vi "_ParseVIFunc.vi"(11 "string":string="VIB(sin(x)+2,VIA(x,y), VIB(z))") -> (0 "valid":bool=TRUE, 2 "Array of Strings":string[](array[string])=["sin(x)+2", "VIA(x", "y)", " VIB(z)"], 3 "before substring":string="VIB")   [LabVIEW 2017]
uses:
  <userlib>/_NEVSTOP/Communicable State Machine(CSM)/Communicable State Machine.lvlib
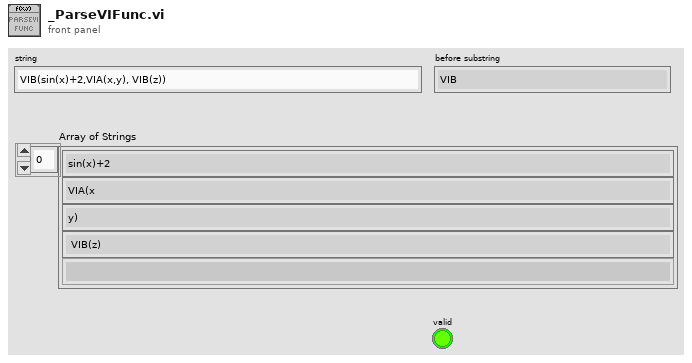
[diagram p1: front panel]
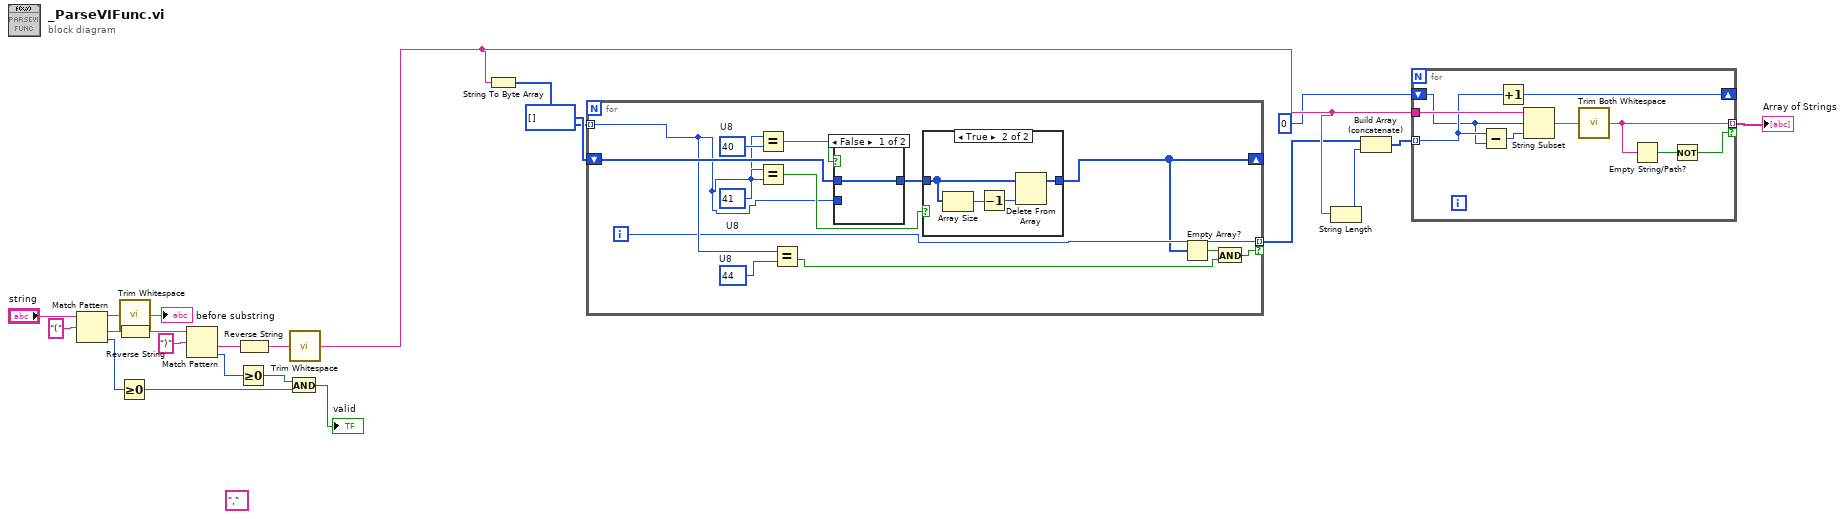
[diagram p0: block diagram]
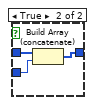
[diagram p3: hidden frame]
diagram:
  (unwired) "," ("regular expression")
  n1 = Match Pattern(string="string", regular expression="(") -> (before substring=w21:string, after substring=w19:string, offset past match=w17:i32)  [unwired: 1 in, 1 out]
  n2 = Greater Or Equal To 0?(x=w17) -> (x >= 0?=w14:bool)
  n3 = call <vilib>:"Trim Whitespace.vi"("string"=w21) -> ("trimmed string"=→"before substring":string)  [unwired: 1 in]
  n4 = Reverse String(1:w19) -> (0:w12:string)
  n5 = Match Pattern(string=w12, regular expression=")") -> (after substring=w11:string, offset past match=w16:i32)  [unwired: 1 in, 2 out]
  n6 = Greater Or Equal To 0?(x=w16) -> (x >= 0?=w15:bool)
  n7 = Reverse String(1:w11) -> (0:w10:string)
  n8 = And(x=w15, y=w14) -> (x .and. y?=→"valid":bool)
  n9 = call <vilib>:"Trim Whitespace.vi"("string"=w10) -> ("trimmed string"=w8:string)  [unwired: 1 in]
  n10 = String To Byte Array(string=w8) -> (unsigned byte array=w6:u8[])
  n11 = for {
    tunnel: w6 -> [w28] mode=indexing
    shift-right: [w25] -> _
    shift-left: i32[] [] -> [w30]
    tunnel: [w27] -> w5 mode=indexing if=w24
    i -> [w27]
    w29 = u8 44  # U8
    w33 = u8 41  # U8
    w35 = u8 40  # U8
    n12 = Equal?(x=w28, y=w35) -> (x = y?=w34:bool)
    n13 = Equal?(x=w33, y=w28) -> (x = y?=w31:bool)
    n14 = Equal?(x=w28, y=w29) -> (x = y?=w23:bool)
    n15 = case shown="False" w34 {
      tunnel: w30 -> [w41 w44]
      tunnel: w28 -> [_ w43]
      tunnel: [w41 w42] -> w32
      frame False {
      }
      frame True {
        n16 = Build Array (concatenate)(w44, w43) -> (w42:i32[])
      }
    }
    n17 = case shown="True" w31 {
      tunnel: w32 -> [w36 w39]
      tunnel: [w36 w37] -> w25
      frame False {
      }
      frame True {
        n18 = Array Size(array=w39) -> (size(s)=w40:i32)
        n19 = Decrement(x=w40) -> (x-1=w38:i32)
        n20 = Delete From Array(array=w39, index=w38) -> (array with subset deleted=w37:i32[])  [unwired: 1 in, 1 out]
      }
    }
    n21 = Empty Array?(array=w25) -> (empty?=w26:bool)
    n22 = And(x=w26, y=w23) -> (x .and. y?=w24:bool)
  }
  n23 = String Length(string=w8) -> (length=w1:i32)
  n24 = Build Array (concatenate)(w5, w1) -> (w2:i32[])
  n25 = for {
    tunnel: w8 -> [w53]
    tunnel: w2 -> [w51] mode=indexing
    tunnel: [w47] -> w3 mode=indexing if=w45
    shift-right: [w48] -> _
    shift-left: 0 ("Numeric") -> [w49]
    n26 = Subtract(x=w51, y=w49) -> (x-y=w50:i32)
    n27 = Increment(x=w51) -> (x+1=w48:i32)
    n28 = String Subset(string=w53, offset (0)=w49, length (rest)=w50) -> (substring=w52:string)
    n29 = call <userlib>:"Trim Both Whitespace.vi"("string"=w52) -> ("trimmed string"=w47:string)  [unwired: 1 in]
    n30 = Empty String/Path?(string/path=w47) -> (empty?=w46:bool)
    n31 = Not(x=w46) -> (.not. x?=w45:bool)
  }
  "Array of Strings" <- w3
